vi "Get Acquisition Regs.vi"(2 "acq":refnum<class "niUSRP Rx DSP v2 FPGA.lvclass">) -> (4 "dsp":T1 caption="misc")   [LabVIEW 2025, in "niUSRP Rx DSP v2 FPGA.lvclass"]
uses:
  niUSRP Rx DSP v2 FPGA.lvclass
  Typedefs/DSP Shared Regs.ctl
  niUSRP Rx DSP v2 FPGA.lvclass/niUSRP Rx DSP v2 FPGA.ctl
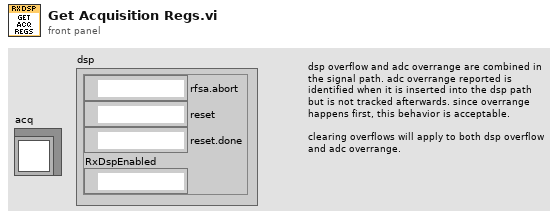
[diagram p1: front panel]
types:
  T1 = typedef "niUSRP Rx DSP v2 FPGA.lvclass/DSP Shared Regs.ctl" = cluster{"rfsa.abort":refnum<k21>, "reset":refnum<k21>, "reset.done":refnum<k21>, "RxDspEnabled":refnum<k21>}
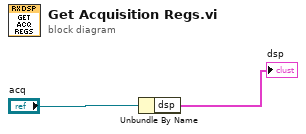
[diagram p0: block diagram]
diagram:
  n1 = Unbundle By Name("acq") -> ("dsp"=→"dsp":T1)
